vi "ReplaceHeader.vi"(0 "In":string, 1 "Size":bool, 5 "string":string, 12 "KEY1":string, 13 "KEY2":string) -> (4 "Out":string, 8 "Size_Out":i32, 10 "StartPos":i32)   [LabVIEW 2017]
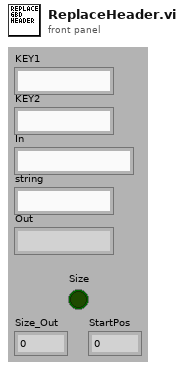
[diagram p1: front panel]
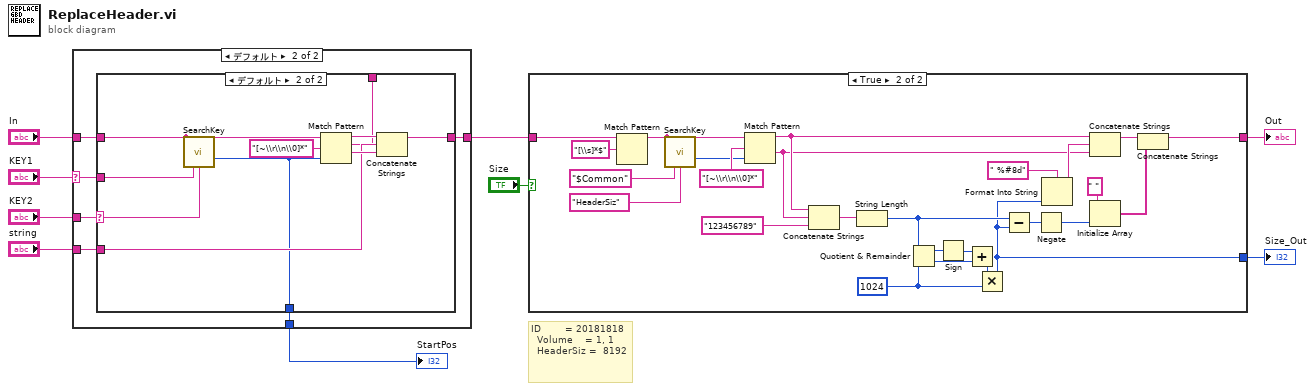
[diagram p0: block diagram]
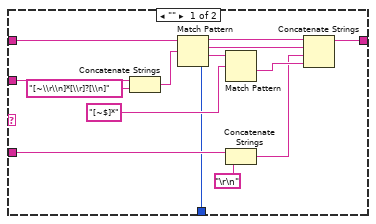
[diagram p3: hidden frame]
diagram:
  # "ID        = 20181818\n  Volume    = 1, 1\n  HeaderSiz =  8192"
  n1 = case shown="デフォルト" "KEY1" {
    selector: "KEY1" -> [_ w12]
    tunnel: "In" -> [w10 w16]
    tunnel: "string" -> [_ w15]
    tunnel: [w10 w14] -> w7
    tunnel: "KEY2" -> [_ w13]
    tunnel: [_ w11] -> w1
    frame "" {
    }
    frame Default {
      n2 = case shown="デフォルト" w13 {
        selector: w13 -> [_ w34]
        tunnel: w16 -> [w28 w40]
        tunnel: w12 -> [w27 w36]
        tunnel: w15 -> [w20 w33]
        tunnel: [w21 w35] -> w14
        tunnel: [w17 w32] -> w11
        tunnel: [_ w31] -> _
        frame "" {
          n3 = Concatenate Strings(w27, "[~\\r\\n]*[\\r]?[\\n]" ("string")) -> (w30:string)
          n4 = Match Pattern(string=w28, regular expression=w30) -> (before substring=w24:string, match substring=w23:string, after substring=w26:string, offset past match=w17:i32)  [unwired: 1 out]
          n5 = Match Pattern(string=w26, regular expression="[~$]*" ("string")) -> (after substring=w22:string)  [unwired: 4 out]
          n6 = Concatenate Strings(w20, "\r\n") -> (w19:string)
          n7 = Concatenate Strings(w24, w23, w19, w22) -> (w21:string)
        }
        frame Default {
          n8 = call "SearchKey.vi"("In"=w40, "KEY1"=w36, "KEY2"=w34) -> ("Position"=w32:i32)  [unwired: 12 out]
          n9 = Match Pattern(string=w40, regular expression="[~\\r\\n\\0]*" ("string"), offset (0)=w32) -> (before substring=w38:string, match substring=w31:string, after substring=w37:string)  [unwired: 1 out]
          n10 = Concatenate Strings(w38, w33, w37) -> (w35:string)
        }
      }
    }
  }
  "StartPos" <- w1
  n11 = case shown="TRUE" "Size" {
    tunnel: w7 -> [w41 w59]
    tunnel: [w41 w60] -> w6
    tunnel: [_ w49] -> w4
    frame False {
    }
    frame True {
      w61 = 1024 ("y")
      n12 = Match Pattern(string=w59, regular expression="[\\s]*$") -> (before substring=w51:string)  [unwired: 4 out]
      n13 = call "SearchKey.vi"("In"=w51, "KEY1"="$Common", "KEY2"="HeaderSiz" ("KEY1")) -> ("Position"=w50:i32)  [unwired: 12 out]
      n14 = Match Pattern(string=w51, regular expression="[~\\r\\n\\0]*" ("string"), offset (0)=w50) -> (before substring=w45:string, after substring=w44:string)  [unwired: 2 out]
      n15 = Concatenate Strings(w45, w44, "123456789") -> (w42:string)
      n16 = String Length(string=w42) -> (length=w64:i32)
      n17 = Quotient & Remainder(x=w64, y=w61) -> (x-y*floor(x/y)=w67:i32, floor(x/y)=w66:i32)
      n18 = Sign(1:w67) -> (0:w65:i32)
      n19 = Add(x=w65, y=w66) -> (x+y=w62:i32)
      n20 = Multiply(x=w62, y=w61) -> (x*y=w49:i32)
      n21 = Subtract(x=w64, y=w49) -> (x-y=w63:i32)
      n22 = Negate(x=w63) -> (-x=w57:i32)
      n23 = Format Into String(format string=" %#8d", w49) -> (resulting string=w48:string)  [unwired: 2 in, 1 out]
      n24 = Concatenate Strings(w45, w48, w44) -> (w47:string)
      n25 = Initialize Array(" ", w57) -> (w56:string[])
      n26 = Concatenate Strings(w47, w56) -> (w60:string)
    }
  }
  "Out" <- w6
  "Size_Out" <- w4
